vi "Read Config Data.vi"(8 "Error In":errorcluster, 11 "configuration file in":path) -> (0 "Error Out":errorcluster, 2 "Hardware Settings":T1={"AI Voltage Channel"="PCI-6221/ai0:3", "Sample Rate (Hz)"=1000.0, "Samples per channel"=1000, "AO Voltage Channel"="PCI-6221/ao1"}, 3 "configuration file out":path)   [LabVIEW 2019]
uses:
  Hardware Settings.ctl
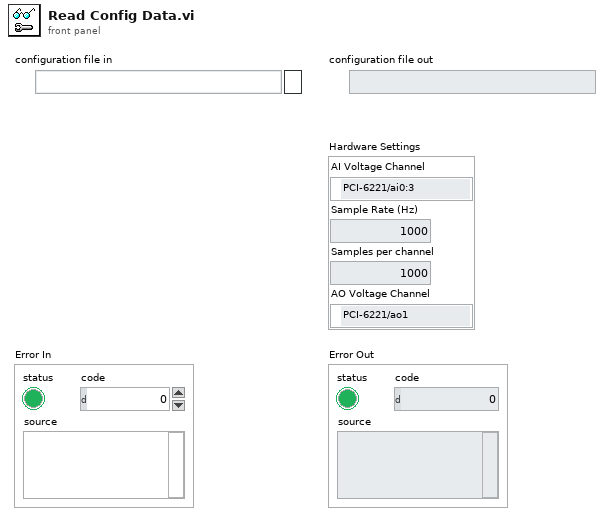
[diagram p1: front panel]
types:
  T1 = typedef "Hardware Settings.ctl" = cluster{"AI Voltage Channel":tag, "Sample Rate (Hz)":dbl, "Samples per channel":i32, "AO Voltage Channel":tag}
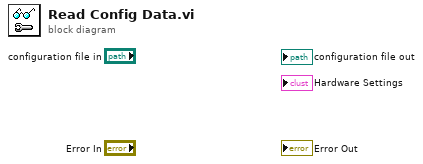
[diagram p0: block diagram]
diagram:
